vi "Format Instrument String Command.vi"(8 "error in (no error)":errorcluster, 9 "MetaData Lookup in":variant, 10 "MetaData":dbl[](array[numeric]), 11 "Command Parameters":T1) -> (0 "error out":errorcluster, 1 "MetaData Lookup out":variant, 3 "Command":string)   [LabVIEW 2020, in "Instrument Addon Engine.lvlib"]
uses:
  Instrument Addon Engine.lvlib
  Addon Shared/Types/Command Parameters.ctl
  Addon Shared/Types/Linked Channel Cluster.ctl
  Addon Shared/Types/Meta Data RT Configuration Cluster.ctl
  Addon Shared/Types/MetaData Parameters.ctl
  Addon Shared/Types/Protocol Data Type.ctl
  Addon Shared/Types/Metadata Channel Type.ctl
  Addon Shared/Types/Type Cast Type.ctl
  Addon Shared/Types/Endian.ctl
  Addon Shared/Instrument Addon Shared.lvlib
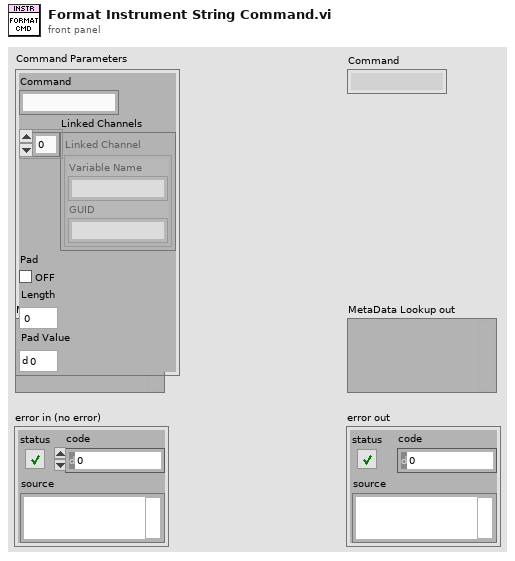
[diagram p1: front panel]
types:
  T1 = typedef "Instrument Addon Shared.lvlib/Command Parameters.ctl" = cluster{"Command":string, "Linked Channels":T2[], "Pad":bool, "Length":u32, "Pad Value":u8}
  T2 = typedef "Instrument Addon Shared.lvlib/Linked Channel Cluster.ctl" = cluster{"Variable Name":string, "GUID":string}
  T3 = typedef "Instrument Addon Shared.lvlib/Meta Data RT Configuration Cluster.ctl" = cluster{"MetaData Parameters":T4, "Data Index":i32, "Data Length":i32}
  T4 = typedef "Instrument Addon Shared.lvlib/MetaData Parameters.ctl" = cluster{"Data Type":T5, "Channel Type":T6, "List":string[], "Format String":string, "Type":T7, "Delimiter":string, "Endian":T8}
  T5 = typedef "Instrument Addon Shared.lvlib/Protocol Data Type.ctl" = enum16{"Single Channel", "Array"}
  T6 = typedef "Instrument Addon Shared.lvlib/Metadata Channel Type.ctl" = enum16{"Enumerated List", "Format", "Type Cast"}
  T7 = typedef "Instrument Addon Shared.lvlib/Type Cast Type.ctl" = enum16{"DBL", "SGL", "U64", "U32", "U16", "U8", "I64", "I32", "I16", "I8"}
  T8 = typedef "Instrument Addon Shared.lvlib/Endian.ctl" = enum16{"Native", "Little", "Big"}
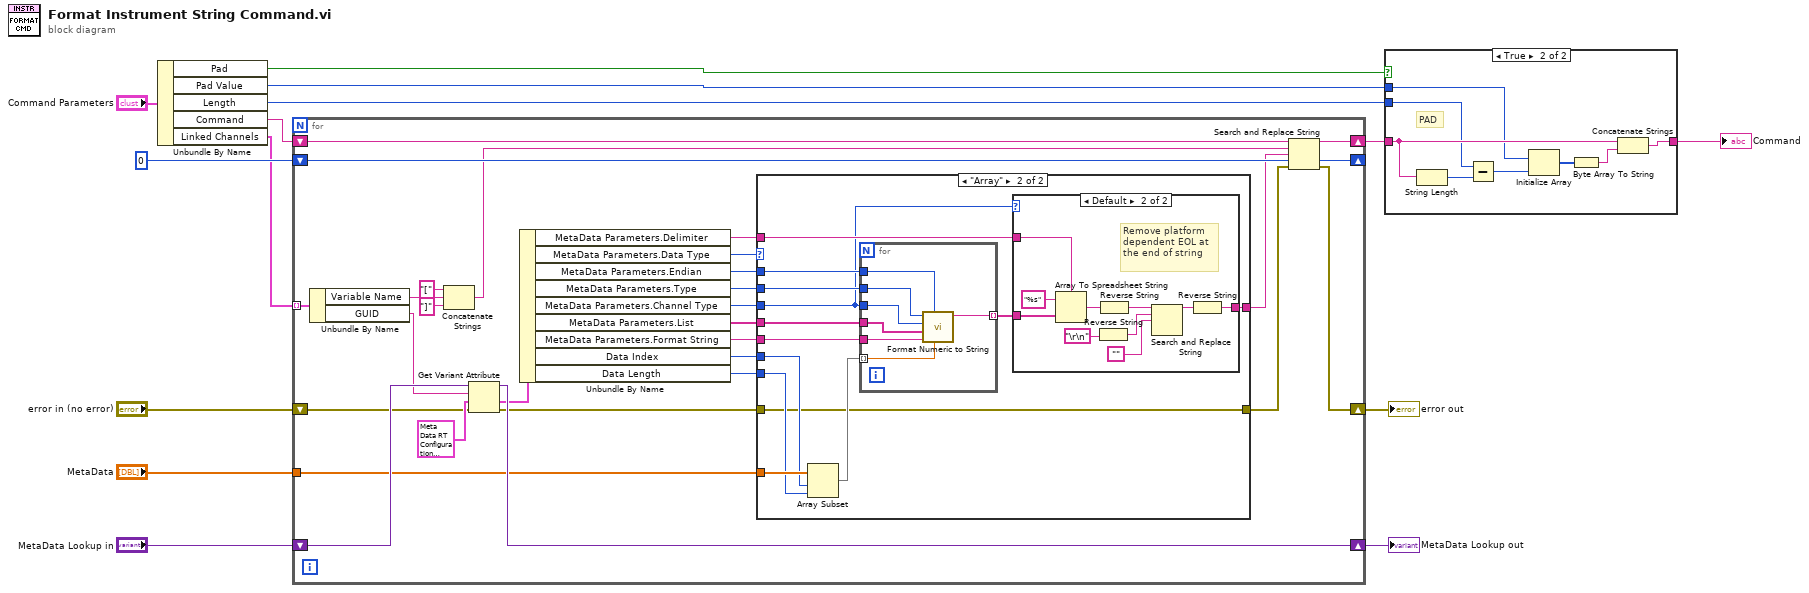
[diagram p0: block diagram]
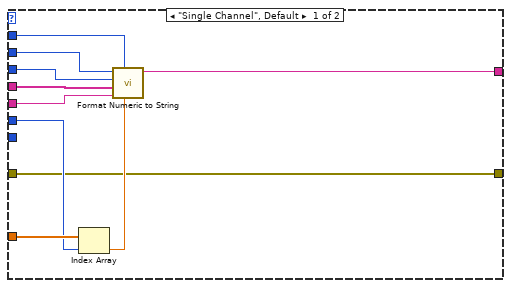
[diagram p3: hidden frame]
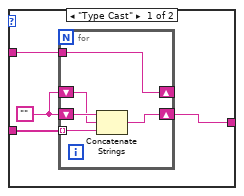
[diagram p4: hidden frame]
diagram:
  n1 = Unbundle By Name("Command Parameters") -> ("Pad"=w2:bool, "Pad Value"=w1:u8, "Length"=w3:u32, "Command"=w11:string, "Linked Channels"=w7:T2[])
  n2 = for {
    tunnel: w7 -> [w43] mode=indexing
    shift-right: [w39] -> w10
    shift-left: "MetaData Lookup in" -> [w42]
    shift-right: [w31] -> w14
    shift-left: "error in (no error)" -> [w40]
    shift-right: [w29] -> w5
    shift-left: w11 -> [w32]
    tunnel: "MetaData" -> [w22]
    shift-right: [w30] -> _
    shift-left: 0 -> [w34]
    n3 = Unbundle By Name(w43) -> ("Variable Name"=w36:string, "GUID"=w24:string)
    n4 = Concatenate Strings("[" ("string"), w36, "]" ("string")) -> (w33:string)
    n5 = Get Variant Attribute(Variant=w42, name=w24, default value (empty Variant)=T3 {"MetaData Parameters"={"Data Type"=enum."Single Channel", "Channel Type"=enum."Enumerated List", "List"=[], "Format String"="", "Type"=enum."DBL", "Delimiter"="", "Endian"=enum."Native"}, "Data Index"=0, "Data Length"=0}, error in=w40) -> (duplicate Variant=w39:variant, value=w38:T3, error out=w16:errorcluster)  [unwired: 1 out]
    n6 = Unbundle By Name(w38) -> ("MetaData Parameters.Delimiter"=w18:string, "MetaData Parameters.Data Type"=w19:T5, "MetaData Parameters.Endian"=w15:T8, "MetaData Parameters.Type"=w23:T7, "MetaData Parameters.Channel Type"=w28:T6, "MetaData Parameters.List"=w26:string[], "MetaData Parameters.Format String"=w27:string, "Data Index"=w21:i32, "Data Length"=w20:i32)
    n7 = case shown="\"Array\"" w19 {
      tunnel: w28 -> [w48 w54]
      tunnel: w27 -> [w50 w66]
      tunnel: w26 -> [w49 w65]
      tunnel: [w46 w56] -> w25
      tunnel: w23 -> [w47 w64]
      tunnel: w22 -> [w53 w63]
      tunnel: w21 -> [w52 w62]
      tunnel: w20 -> [_ w61]
      tunnel: w18 -> [_ w58]
      tunnel: [w45 w57] -> w17
      tunnel: w16 -> [w45 w57]
      tunnel: w15 -> [w44 w55]
      frame "Single Channel", Default {
        n8 = Index Array(array=w53, index=w52) -> (element=w51:dbl)
        n9 = call "Format Numeric to String.vi"("Numeric"=w51, "Endian"=w44, "Format String"=w50, "List"=w49, "Channel Type"=w48, "Type"=w47) -> ("Value"=w46:string)  [unwired: 5 in]
      }
      frame "Array" {
        n10 = Array Subset(array=w63, index=w62, length=w61) -> (w60:dbl[])
        n11 = for {
          tunnel: w54 -> [w92]
          tunnel: w66 -> [w88]
          tunnel: w65 -> [w91]
          tunnel: [w90] -> w59 mode=indexing
          tunnel: w64 -> [w89]
          tunnel: w60 -> [w87] mode=indexing
          tunnel: w55 -> [w86]
          n12 = call "Format Numeric to String.vi"("Numeric"=w87, "Endian"=w86, "Format String"=w88, "List"=w91, "Channel Type"=w92, "Type"=w89) -> ("Value"=w90:string)  [unwired: 5 in]
        }
        n13 = case shown="Default" w54 {
          tunnel: w59 -> [w70 w85]
          tunnel: w58 -> [w67 w84]
          tunnel: [w69 w76] -> w56
          frame "Type Cast" {
            w68 = ""
            n14 = for {
              tunnel: w70 -> [w75] mode=indexing
              shift-right: [w74] -> w69
              shift-left: w68 -> [w73]
              shift-right: [w71] -> _
              shift-left: w68 -> [w72]
              tunnel: w67 -> [w71]
              n15 = Concatenate Strings(w73, w72, w75) -> (w74:string)
            }
          }
          frame Default {
            # "Remove platform dependent EOL at the end of string"
            n16 = Array To Spreadsheet String(delimiter (Tab)=w84, array=w85, 3:"%s" ("format string")) -> (spreadsheet string=w81:string)
            n17 = Reverse String(1:"\r\n" ("End of Line Constant")) -> (0:w79:string)
            n18 = Reverse String(1:w81) -> (0:w80:string)
            n19 = Search and Replace String(input string=w80, search string=w79, replace string="") -> (result string=w77:string)  [unwired: 5 in, 3 out]
            n20 = Reverse String(1:w77) -> (0:w76:string)
          }
        }
      }
    }
    n21 = Search and Replace String(input string=w32, search string=w33, replace string=w25, offset=w34, error in=w17) -> (result string=w29:string, offset past replacement=w30:i32, error out=w31:errorcluster)  [unwired: 3 in, 1 out]
  }
  "error out" <- w14
  "MetaData Lookup out" <- w10
  n22 = case shown="True" w2 {
    tunnel: w5 -> [w93 w98]
    tunnel: [w93 w96] -> w4
    tunnel: w3 -> [_ w95]
    tunnel: w1 -> [_ w94]
    frame False {
    }
    frame True {
      # "PAD"
      n23 = String Length(string=w98) -> (length=w101:i32)
      n24 = Subtract(x=w95, y=w101) -> (x-y=w100:u32)
      n25 = Initialize Array(w94, w100) -> (w99:u8[])
      n26 = Byte Array To String(unsigned byte array=w99) -> (string=w97:string)
      n27 = Concatenate Strings(w98, w97) -> (w96:string)
    }
  }
  "Command" <- w4
